vi "Test2.vi"(10 "B":i32, 11 "A":i32) -> (2 "D":i32, 3 "C":i32)   [LabVIEW 2017]
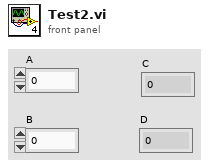
[diagram p1: front panel]
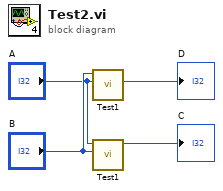
[diagram p0: block diagram]
diagram:
  n1 = call "Test1.vi"("B"="A", "A"="B") -> ("D"=→"D":i32)  [unwired: 8 in, 1 out]
  n2 = call "Test1.vi"("B"="B", "A"="A") -> ("C"=→"C":i32)  [unwired: 8 in, 1 out]
